vi "SJ_Phase_Average_LDA.vi"(8 "Transpose? (False)":bool, 9 "No. of Bins":i32=30, 11 "1D Signal":dbl[](array[numeric])=[0.5040180756789142, 0.4920161135872081, 0.4139706571157036, 0.3514761512703959, 0.328013137284893, 0.24429776847397908, 0.17464927129376565, 0.13300957289690787, 0.12898616487426454, 0.10153973918608236, 0.17036966727768935, 0.20756788855682703, 0.2925978323950259, 0.3754927061879243, 0.4712919934451292, 0.5161336574985805, 0.5688922326713383, 0.6041348031076303, 0.617170268610945, 0.5314312057713051, 0.5040180756789142, 0.38907291400217214, 0.27783539358252807, 0.2053221786995407, 0.14729685098365844, 0.19642555608031134, 0.2419575114773357, 0.3594158549457278, 0.5688922326713383, 0.4830959307395156, 0.5283631675233643, 0.5161336574985805, 0.3973140759846684, 0.386348178544617, 0.3647473436891949, 0.2419575114773357, 0.20086081848710216, 0.15977857793083036, 0.13909712890547168, 0.12698864379669558, 0.16611587118083812, 0.18545638550824353, 0.26330231288553463, 0.34097731625809025, 0.44227483396003364, 0.5161336574985805, 0.5688922326713383, 0.4920161135872081, 0.5879961845969328, 0.54690720136361, 0.42238614698923793, 0.3945558255861209, 0.2657021929248762, 0.18328606946593842, 0.17464927129376565, 0.18328606946593842, 0.2419575114773357, 0.32543349096689256, 0.4596008249034499, 0.47717984660981494, 0.5161336574985805, 0.4920161135872081, 0.49501294678819174, 0.5009999347085525, 0.3383757343267596, 0.2657021929248762, 0.20756788855682703, 0.12499743496167756, 0.20309343352844164, 0.12499743496167756, 0.11707727251584568, 0.18982661424727823, 0.3754927061879243, 0.3514761512703959, 0.41957840373935784, 0.4830959307395156, 0.5283631675233643, 0.5376030407230764, 0.5376030407230764, 0.5376030407230764, 0.4596008249034499, 0.3620843845987681, 0.27783539358252807, 0.2280218862894465, 0.14113272259311518, 0.19642555608031134, 0.2537469047748594, 0.3076136738414226, 0.44227483396003364, 0.5407069136943436, 0.49501294678819174, 0.49800291146809295, 0.49800291146809295, 0.37010628093393316, 0.3754927061879243, 0.27783539358252807, 0.18982661424727823, 0.14729685098365844, 0.1131551041103975, 0.13099938201800645, 0.13099938201800645, 0.20756788855682703, 0.26089789622788107, 0.328013137284893, 0.439418361134121, 0.49800291146809295, 0.553150616483236, 0.5847991458946908, 0.5879961845969328, 0.49501294678819174, 0.45379743188287025, 0.3973140759846684, 0.3126729231107592, 0.19642555608031134, 0.17036966727768935, 0.19422283761779593, 0.22113773189777267, 0.3620843845987681, 0.47717984660981494, 0.5130870163984499, 0.5594227441359473, 0.5222341522265641, 0.44227483396003364, 0.3754927061879243, 0.32543349096689256, 0.2419575114773357, 0.19642555608031134, 0.16823458805776845, 0.13503552964041518, 0.12102470196956819, 0.1767937462859607, 0.1639937103270598, 0.2802752597608067, 0.3567665733319275, 0.4111707088100722, 0.5376030407230764, 0.5222341522265641, 0.6806593256678739, 0.5976606166642047, 0.5161336574985805, 0.456702380381403, 0.4252008231140979, 0.3126729231107592, 0.23032261247397698, 0.19642555608031134, 0.15977857793083036, 0.2537469047748594, 0.343597888571441, 0.41957840373935784, 0.5100616448302553, 0.5130870163984499, 0.4860576433912698, 0.46835181194042763, 0.462506265335099, 0.343597888571441, 0.23728589099600736, 0.17036966727768935, 0.1131551041103975, 0.13300957289690787, 0.11119893762224128, 0.13503552964041518, 0.20309343352844164, 0.2681199702040179, 0.31014581616483516, 0.4509129973389887, 0.465432332477576, 0.5040180756789142, 0.5879961845969328, 0.5847991458946908, 0.5407069136943436, 0.4920161135872081, 0.4167645168429057, 0.2975761685548989, 0.23032261247397698, 0.1639937103270598, 0.17464927129376565, 0.25851130457401084, 0.3203065706710776, 0.3594158549457278, 0.49800291146809295, 0.5100616448302553, 0.49501294678819174, 0.4480221145394636, 0.386348178544617, 0.34097731625809025, 0.28764638704882295, 0.18328606946593842, 0.16823458805776845, 0.13099938201800645, 0.12499743496167756, 0.13099938201800645, 0.19201635023504324, 0.2280218862894465, 0.386348178544617, 0.43655555119421463, 0.49800291146809295, 0.5688922326713383, 0.5657236226361149, 0.5752363428117551, 0.5784117852792484, 0.49501294678819174, 0.4280356383708891, 0.31775922348005836, 0.18328606946593842, 0.16188784132848047, 0.17250125282973547, 0.18982661424727823, 0.2975761685548989, 0.4139706571157036, 0.44227483396003364, 0.5009999347085525, 0.5222341522265641, 0.44227483396003364, 0.4028385324386853, 0.367429624643002, 0.26089789622788107, 0.18111211000632868, 0.14935793152538465, 0.11119893762224128, 0.13099938201800645, 0.12300327266484071, 0.18328606946593842, 0.24429776847397908, 0.35411177515287573, 0.3918173044534722, 0.5100616448302553, 0.5345207418649437, 0.5912154103030958, 0.5784117852792484, 0.5438034923271824, 0.5009999347085525, 0.383617628329213, 0.29508943888607275, 0.22342942043349298, 0.13705841140090327, 0.15768553598177495, 0.20309343352844164, 0.3203065706710776, 0.38907291400217214, 0.4890402845665881, 0.519173232085027, 0.49501294678819174, 0.47717984660981494, 0.37010628093393316, 0.3331808304879178, 0.2561202282498407, 0.19864509695357882, 0.12898616487426454, 0.13300957289690787, 0.13099938201800645, 0.13099938201800645, 0.18111211000632868, 0.25851130457401084, 0.31775922348005836, 0.37010628093393316, 0.49501294678819174, 0.54690720136361, 0.5562903990373093, 0.5879961845969328, 0.6435751025127421, 0.474225531300315, 0.37010628093393316, 0.3076136738414226, 0.23032261247397698, 0.16188784132848047, 0.14729685098365844, 0.23961295072023112, 0.31014581616483516, 0.4083907130756498, 0.5100616448302553, 0.5345207418649437, 0.5407069136943436, 0.5009999347085525, 0.4139706571157036, 0.328013137284893, 0.2802752597608067, 0.18111211000632868, 0.13909712890547168, 0.2053221786995407, 0.12698864379669558, 0.13300957289690787, 0.16823458805776845, 0.2419575114773357, 0.31775922348005836, 0.4083907130756498, 0.5100616448302553, 0.5562903990373093, 0.6041348031076303, 0.6041348031076303, 0.5784117852792484, 0.4830959307395156, 0.3918173044534722, 0.4028385324386853, 0.22571701040555106, 0.19864509695357882, 0.17250125282973547, 0.20980967790269592, 0.2975761685548989, 0.4280356383708891, 0.456702380381403, 0.5161336574985805, 0.5130870163984499, 0.4252008231140979, 0.3331808304879178, 0.31520676134106485, 0.2681199702040179, 0.18982661424727823, 0.17036966727768935, 0.11119893762224128, 0.11904322623994792, 0.11510846206791445, 0.17464927129376565, 0.24664461631553988, 0.328013137284893, 0.4056046837298525, 0.49800291146809295, 0.5500325989778979, 0.5688922326713383, 0.5688922326713383, 0.5816092994930254, 0.4920161135872081, 0.42238614698923793, 0.328013137284893, 0.2419575114773357, 0.20309343352844164, 0.14113272259311518, 0.21658473602406855, 0.30510004596689144, 0.3973140759846684, 0.4890402845665881, 0.5070292634594806, 0.43655555119421463, 0.465432332477576, 0.4056046837298525, 0.3357688239451295, 0.29012452181270276, 0.22113773189777267, 0.15768553598177495, 0.10538638011916049, 0.11119893762224128, 0.12102470196956819, 0.19422283761779593, 0.24900907294131921, 0.3488350647169022, 0.3620843845987681, 0.4860576433912698, 0.553150616483236, 0.6204396597878676, 0.610638007733154, 0.553150616483236, 0.553150616483236, 0.40006640240191405, 0.3331808304879178, 0.2419575114773357, 0.16188784132848047, 0.17250125282973547, 0.2280218862894465, 0.2802752597608067, 0.4056046837298525, 0.4056046837298525, 0.5100616448302553, 0.5040180756789142, 0.465432332477576, 0.4028385324386853, 0.35411177515287573, 0.27783539358252807, 0.21206850319442536, 0.15143505793601933, 0.12698864379669558, 0.11707727251584568, 0.15143505793601933, 0.19642555608031134, 0.2537469047748594, 0.35411177515287573, 0.3973140759846684, 0.46835181194042763, 0.5688922326713383, 0.5816092994930254, 0.7012664582352968, 0.5720532902666493, 0.5100616448302553, 0.4167645168429057, 0.328013137284893, 0.22342942043349298, 0.13503552964041518, 0.1555891490978629, 0.16823458805776845, 0.31014581616483516, 0.4111707088100722, 0.4509129973389887, 0.4830959307395156, 0.519173232085027, 0.47717984660981494, 0.41957840373935784, 0.37010628093393316, 0.25851130457401084, 0.19864509695357882, 0.17036966727768935, 0.12102470196956819, 0.11119893762224128, 0.15977857793083036, 0.20980967790269592, 0.24429776847397908, 0.2419575114773357, 0.4056046837298525, 0.45379743188287025, 0.474225531300315, 0.5594227441359473, 0.5562903990373093, 0.5562903990373093, 0.4920161135872081, 0.40006640240191405, 0.30510004596689144, 0.2513691484700872, 0.18982661424727823, 0.13705841140090327, 0.22571701040555106, 0.31014581616483516, 0.4083907130756498, 0.5252879490451223, 0.5625769308355976, 0.5161336574985805, 0.4509129973389887, 0.4280356383708891, 0.3567665733319275, 0.28764638704882295, 0.22571701040555106, 0.16823458805776845, 0.14935793152538465, 0.1131551041103975, 0.13099938201800645, 0.16823458805776845, 0.2537469047748594, 0.31775922348005836, 0.4111707088100722, 0.439418361134121, 0.5500325989778979, 0.54690720136361, 0.5688922326713383, 0.5720532902666493, 0.5161336574985805, 0.4280356383708891, 0.35411177515287573, 0.2561202282498407, 0.17895472484035338, 0.1639937103270598, 0.20309343352844164, 0.3514761512703959, 0.4252008231140979, 0.5376030407230764, 0.5130870163984499, 0.5283631675233643, 0.5161336574985805, 0.37010628093393316, 0.3488350647169022, 0.25851130457401084, 0.1876331596475089, 0.17464927129376565, 0.13705841140090327, 0.060881483864868496, 0.14318422198536215, 0.1639937103270598, 0.21206850319442536, 0.27783539358252807, 0.3488350647169022, 0.45379743188287025, 0.5500325989778979, 0.553150616483236, 0.5562903990373093, 0.5562903990373093, 0.4860576433912698, 0.41957840373935784, 0.328013137284893, 0.21658473602406855, 0.18111211000632868, 0.1639937103270598, 0.18328606946593842, 0.2753908342994117, 0.4139706571157036, 0.4712919934451292, 0.47717984660981494, 0.54690720136361, 0.3567665733319275, 0.41957840373935784, 0.4280356383708891, 0.26089789622788107, 0.23264069619599106, 0.18111211000632868, 0.14318422198536215, 0.11707727251584568, 0.13503552964041518, 0.18328606946593842, 0.2419575114773357, 0.3025814356719517, 0.3594158549457278, 0.465432332477576, 0.5376030407230764, 0.5752363428117551, 0.5879961845969328, 0.5500325989778979, 0.5161336574985805, 0.456702380381403, 0.343597888571441, 0.2513691484700872, 0.2053221786995407, 0.14523254861140902, 0.20756788855682703, 0.3331808304879178, 0.3594158549457278, 0.4509129973389887, 0.54690720136361, 0.5070292634594806, 0.4830959307395156, 0.4280356383708891, 0.3126729231107592, 0.28272179232406114, 0.23032261247397698, 0.18982661424727823, 0.13705841140090327, 0.12898616487426454, 0.153508913337103, 0.18328606946593842, 0.23728589099600736, 0.3126729231107592, 0.3918173044534722, 0.44227483396003364, 0.5161336574985805, 0.6402547993835251, 0.5161336574985805, 0.6073751962965519, 0.519173232085027, 0.4111707088100722, 0.3331808304879178, 0.3228726149025192, 0.18982661424727823, 0.1639937103270598, 0.18545638550824353, 0.27053315880959783, 0.40006640240191405, 0.4712919934451292, 0.49800291146809295, 0.4920161135872081, 0.4480221145394636, 0.42238614698923793, 0.3620843845987681, 0.29508943888607275, 0.21886325772961687, 0.1639937103270598, 0.153508913337103, 0.12898616487426454, 0.14113272259311518, 0.17036966727768935, 0.2681199702040179, 0.2925978323950259, 0.37280233299385446, 0.430864227254143, 0.5161336574985805, 0.5314312057713051, 0.5976606166642047, 0.6041348031076303, 0.47717984660981494, 0.4056046837298525, 0.343597888571441, 0.2419575114773357, 0.18111211000632868, 0.17036966727768935, 0.17250125282973547, 0.2802752597608067, 0.4252008231140979, 0.439418361134121, 0.4920161135872081, 0.5040180756789142, 0.4712919934451292, 0.4480221145394636, 0.3945558255861209, 0.2975761685548989, 0.23728589099600736, 0.19201635023504324, 0.15768553598177495, 0.12698864379669558, 0.12300327266484071, 0.16611587118083812, 0.26330231288553463, 0.29508943888607275, 0.37820254913807394, 0.4920161135872081, 0.5070292634594806, 0.5562903990373093, 0.5976606166642047, 0.5847991458946908, 0.5345207418649437, 0.45379743188287025, 0.31520676134106485, 0.23961295072023112, 0.19422283761779593, 0.14318422198536215, 0.17250125282973547, 0.29012452181270276, 0.40006640240191405, 0.46835181194042763]) -> (1 "Variance":dbl[](array[numeric])=[0.0005224809903412037, 0.0005501699701469001, 0.0014543766325612218, 0.00155233345260931, 0.0007763189121830512, 0.0003533585911738399, 0.00041370746932808554, 0.00046282877766196773, 0.0006979112861757282, 0.00025236218015322974, 0.0003248737273189588, 0.00023123591646363978, 0.0010691116871452346, 0.0011922115178257624, 0.0010944029570351822, 0.0008613410505781576, 0.00066335990110124, 0.0016946807517237144, 0.0013350942226953216, 0.0011341471132600897, 0.0009085562430912675, 0.0005921045408061942, 0.0009366838582840715, 0.0009001934747714769, 0.0004842916491997269, 0.00032368809170027734, 0.0008383718187408589, 0.0007431210094132716, 0.0019919795381932556, 0.0012391498634676487], 2 "Standard Deviation":dbl[](array[numeric])=[0.022857843081559633, 0.023455702294898358, 0.038136290230713604, 0.03939966310273871, 0.02786250010647019, 0.018797834746955296, 0.02033980012999355, 0.021513455735003795, 0.026418010640010883, 0.015885911373076135, 0.018024253863030193, 0.015206443254871922, 0.032697273390073896, 0.03452841609205036, 0.033081761697877916, 0.02934861241316457, 0.02575577413127472, 0.041166500357981785, 0.03653894118191332, 0.033677100725271615, 0.030142266721188495, 0.024333198326693395, 0.030605291344538307, 0.03000322440624469, 0.02200662739266803, 0.017991333794365478, 0.028954651072683624, 0.027260245952912304, 0.044631597979382896, 0.03520156052602851], 3 "Phase Averaged Signal":dbl[](array[numeric])=[0.5143441839151416, 0.5063364452861989, 0.4571436284323826, 0.40487799196765223, 0.35117026303946897, 0.26855051090042104, 0.20189978880584278, 0.15759202574722733, 0.1387679547165846, 0.1182663445192635, 0.13943069603298458, 0.18462741785797787, 0.25918269522569204, 0.3255151918457039, 0.40371843955931086, 0.48297768886504155, 0.5387713424380128, 0.5769103674800241, 0.586036268084601, 0.5624893085049238, 0.4919149292197891, 0.40863710538833287, 0.3189805647973408, 0.2311843404982242, 0.17368704818646422, 0.1655910932935557, 0.21381825244352887, 0.31253521410196206, 0.42064065320439176, 0.4814964760093088])   [LabVIEW 2011]
uses:
  <vilib>/Analysis/NI_AALBase.lvlib
panel:
  out "Waveform Graph 3":dbl[][](graph)
  out "Waveform Graph 2":dbl[](graph)
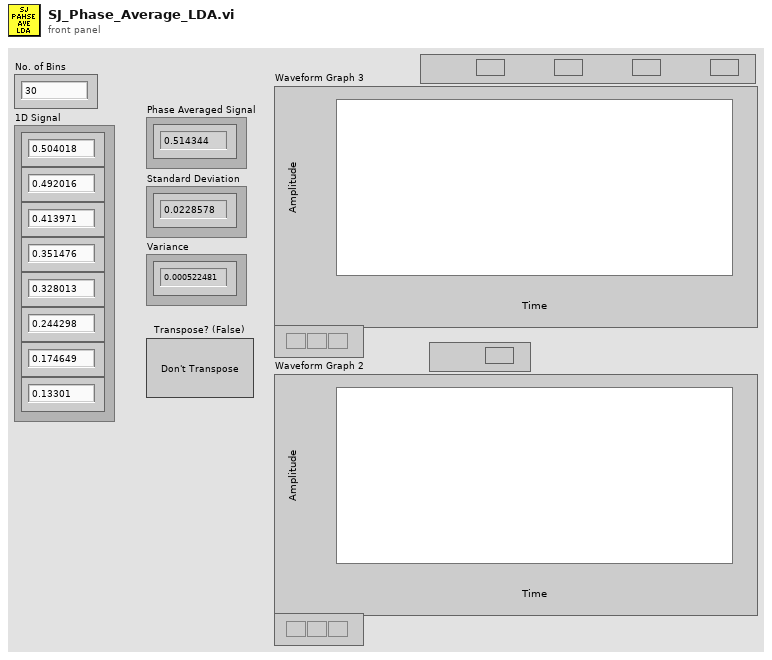
[diagram p1: front panel]
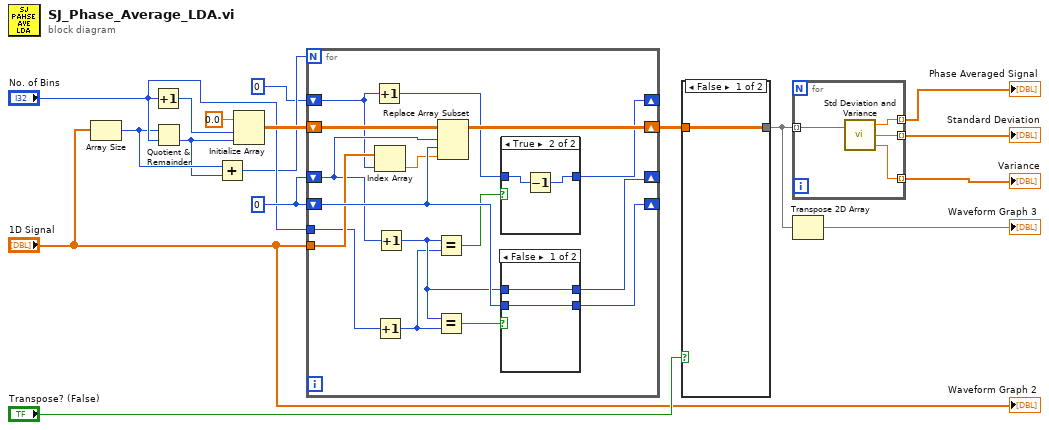
[diagram p0: block diagram]
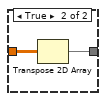
[diagram p2: hidden frame]
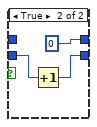
[diagram p4: hidden frame]
diagram:
  w15 = 0
  n1 = Array Size(array="1D Signal") -> (size(s)=w6:i32)
  n2 = Increment(x="No. of Bins") -> (x+1=w7:i32)
  n3 = Quotient & Remainder(x=w6, y="No. of Bins") -> (floor(x/y)=w4:i32)  [unwired: 1 out]
  n4 = Add(x=w6, y=w4) -> (x+y=w5:i32)
  n5 = Initialize Array(0.0 ("cycles"), w7, w4) -> (w16:dbl[][])
  n6 = for {
    N: w5 -> [_]
    tunnel: "1D Signal" -> [w29]
    shift-right: [w32] -> _
    shift-left: w15 -> [w27]
    shift-right: [w31] -> _
    shift-left: w15 -> [w30]
    tunnel: "No. of Bins" -> [w19]
    shift-right: [w25] -> w10
    shift-left: w16 -> [w33]
    shift-right: [w21] -> _
    shift-left: 0 -> [w26]
    n7 = Increment(x=w26) -> (x+1=w20:i32)
    n8 = Index Array(array=w29, index=w26) -> (element=w28:dbl)
    n9 = Increment(x=w19) -> (x+1=w18:i32)
    n10 = Increment(x=w27) -> (x+1=w23:i32)
    n11 = Equal?(x=w23, y=w18) -> (x = y?=w22:bool)
    n12 = Equal?(x=w23, y=w18) -> (x = y?=w24:bool)
    n13 = Replace Array Subset(array=w33, new element=w28, index (row)=w27, index (col)=w30) -> (w25:dbl[][])
    n14 = case shown="True" w22 {
      tunnel: [w34 w35] -> w21
      tunnel: w20 -> [w34 w36]
      frame False {
      }
      frame True {
        n15 = Decrement(x=w36) -> (x-1=w35:i32)
      }
    }
    n16 = case shown="False" w24 {
      tunnel: [w37 0] -> w32
      tunnel: w23 -> [w37 _]
      tunnel: [w38 w40] -> w31
      tunnel: w30 -> [w38 w41]
      frame False {
      }
      frame True {
        n17 = Increment(x=w41) -> (x+1=w40:i32)
      }
    }
  }
  n18 = case shown="False" "Transpose? (False)" {
    tunnel: [w42 w43] -> w1
    tunnel: w10 -> [w42 w44]
    frame False {
    }
    frame True {
      n19 = Transpose 2D Array(2D array=w44) -> (transposed array=w43:dbl[][])
    }
  }
  n20 = for {
    tunnel: w1 -> [w48] mode=indexing
    tunnel: [w47] -> w11 mode=indexing
    tunnel: [w46] -> w13 mode=indexing
    tunnel: [w45] -> w12 mode=indexing
    n21 = call <vilib>:"Std Deviation and Variance.vi"("X"=w48) -> ("mean"=w47:dbl, "standard deviation"=w46:dbl, "variance"=w45:dbl)  [unwired: 1 in]
  }
  "Phase Averaged Signal" <- w11
  "Variance" <- w12
  "Standard Deviation" <- w13
  n22 = Transpose 2D Array(2D array=w1) -> (transposed array=→"Waveform Graph 3":dbl[][])
  "Waveform Graph 2" <- "1D Signal"
